vi "VNA Driver Test.vi"() -> ()   [LabVIEW 2011]
uses:
  VNA Command.ctl
  VNA Driver Ref.ctl
panel:
  in  "Tab Control":enum32{"Stimulus", "Measurements"}(tab)=enum."Measurements"
  out "Get Stimulus":T1
  in  "get stimulus":bool
  in  "set stimulus":bool
  in  "Set Stimulus":T1
  in  "mag":bool=TRUE
  out "plot":cluster{dbl, dbl, dbl[][]}(graph)
  in  "S to Meas":enum32{"S11", "S21", "S12", "S22"}[](array[ring])=[enum."S11"]
  in  "measure":bool
  in  "preset":bool
  in  "config":bool
  in  "init":bool
  in  "VNA Drivers":u16(ring) items=["Agilent VNA", "Summitek VNA"]
  in  "load":bool
  in  "stop":bool
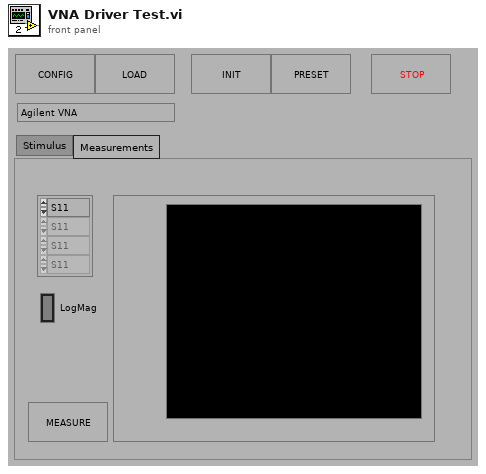
[diagram p1: front panel]
types:
  T1 = cluster{"Use Instrument Settings":bool, "Sweep Type":enum32{"Linear", "Log", "List", "Power", "CW"}, "Sweep":cluster{"Fstart, MHz":dbl, "Fstop, MHz":dbl, "Points":i32}[], "Advanced Settings":bool, "Blank Frequencies":bool, "Power, dBm":dbl, "IFBW, Hz":dbl, "Sweep Time, s":dbl}
  T2 = typedef "VNA Driver Ref.ctl" = refnum<vi>
  T3 = typedef "VNA Command.ctl" = enum16{"LOAD", "INITIALIZE", "PRESET", "GET STIMULUS", "SET STIMULUS", "GET CALIBRATION", "CALIBRATE", "RESTORE", "MEASURE", "RELEASE", "UNLOAD", "CONFIRM", "SORT"}
  T4 = typedef "SP Data.ctl" = cluster{"F0":dbl, "dF":dbl, "Data":cdb[][]}
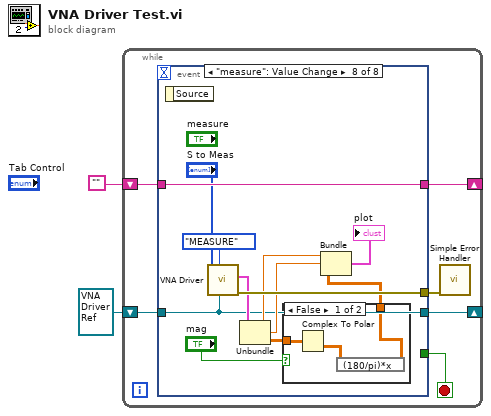
[diagram p0: block diagram]
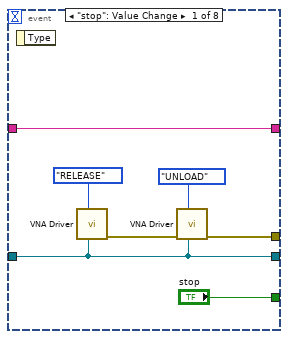
[diagram p2: hidden frame]
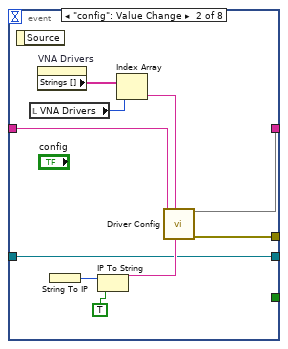
[diagram p3: hidden frame]
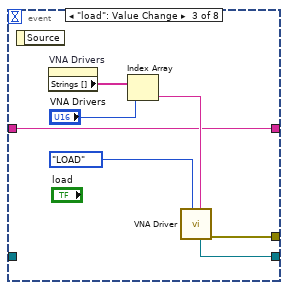
[diagram p4: hidden frame]
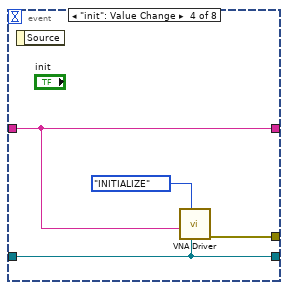
[diagram p5: hidden frame]
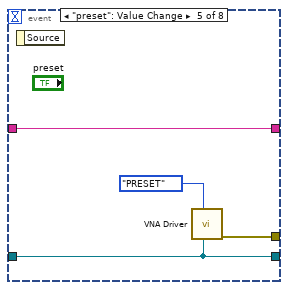
[diagram p6: hidden frame]
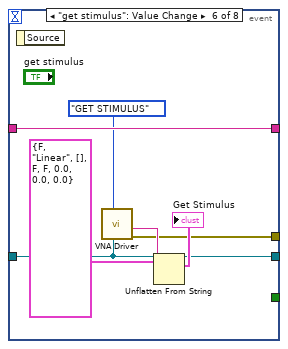
[diagram p7: hidden frame]
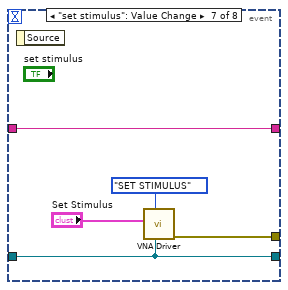
[diagram p8: hidden frame]
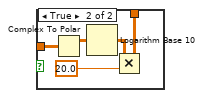
[diagram p9: hidden frame]
diagram:
  n1 = while {
    shift-right: [w6] -> _
    shift-left: "" -> [w5]
    shift-right: [w3] -> _
    shift-left: T2 refnum ("Driver Ref") -> [w4]
    stop <- w8 stop-if-true
    n2 = event shown="[7] \"measure\": Value Change" {
      selector: _ -> [_ _ _ _ _ _ _ _]
      dyn-events: _ -> [_ _ _ _ _ _ _ _]
      timeout: _ -> [_ _ _ _ _ _ _ _]
      tunnel: ["stop" _ _ _ _ _ _ _] -> w8
      tunnel: [w11 w25 w28 w36 w40 w43 w50 w62] -> w7
      tunnel: [w14 w24 w27 w34 w39 w47 w52 w64] -> w6
      tunnel: w5 -> [w14 w23 w27 w34 w39 w47 w52 w64]
      tunnel: w4 -> [w9 w16 _ w33 w37 w41 w48 w53]
      tunnel: [w9 w16 w26 w33 w37 w41 w48 w53] -> w3
      event "stop": Value Change {
        n3 = event-data() -> ()  [unwired: 1 in, 1 out]
        n4 = call "VNA Driver.vi"("Drv Refnum"=w9, "VNA Command"=VNA_Command."RELEASE") -> ("error out"=w12:errorcluster)  [unwired: 5 in, 4 out]
        n5 = call "VNA Driver.vi"("Drv Refnum"=w9, "VNA Command"=VNA_Command."UNLOAD", "error in (no error)"=w12) -> ("error out"=w11:errorcluster)  [unwired: 4 in, 4 out]
      }
      event "config": Value Change {
        n6 = event-data() -> ()  [unwired: 1 in, 1 out]
        n7 = local read "VNA Drivers"() -> (w19:u16)
        n8 = property on="VNA Drivers" class="Ring (strict)"() -> ("Strings []"=w18:string[])  [unwired: 2 in, 2 out]
        n9 = String To IP() -> (0:w22:u32)  [unwired: 1 in]
        n10 = IP To String(1:TRUE, 2:w22) -> (0:w21:string)
        n11 = Index Array(array=w18, index=w19) -> (element=w17:string)
        n12 = call "Driver Config.vi"("CalDue"=w21, "DriverType (\"\")"=w17, "TestStation Client (\"\")"=w23) -> ("error out"=w25:errorcluster, 3:w24)  [unwired: 4 in, 3 out]
      }
      event "load": Value Change {
        n13 = event-data() -> ()  [unwired: 1 in, 1 out]
        n14 = property on="VNA Drivers" class="Ring (strict)"() -> ("Strings []"=w31:string[])  [unwired: 2 in, 2 out]
        n15 = Index Array(array=w31, index="VNA Drivers") -> (element=w29:string)
        n16 = call "VNA Driver.vi"("VNA Driver or\nVNA Configuration (\"\")"=w29, "VNA Command"=VNA_Command."LOAD") -> ("error out"=w28:errorcluster, "dup Drv Refnum"=w26:T2)  [unwired: 5 in, 3 out]
      }
      event "init": Value Change {
        n17 = event-data() -> ()  [unwired: 1 in, 1 out]
        n18 = call "VNA Driver.vi"("Drv Refnum"=w33, "VNA Command"=VNA_Command."INITIALIZE", "Miscellaneous Parameters"=w34) -> ("error out"=w36:errorcluster)  [unwired: 4 in, 4 out]
      }
      event "preset": Value Change {
        n19 = event-data() -> ()  [unwired: 1 in, 1 out]
        n20 = call "VNA Driver.vi"("Drv Refnum"=w37, "VNA Command"=VNA_Command."PRESET") -> ("error out"=w40:errorcluster)  [unwired: 5 in, 4 out]
      }
      event "get stimulus": Value Change {
        n21 = event-data() -> ()  [unwired: 1 in, 1 out]
        n22 = call "VNA Driver.vi"("Drv Refnum"=w41, "VNA Command"=VNA_Command."GET STIMULUS") -> ("error out"=w43:errorcluster, "VNA Flat Output"=w45:string)  [unwired: 5 in, 3 out]
        n23 = Unflatten From String(type=T1 {"Use Instrument Settings"=FALSE, "Sweep Type"=enum."Linear", "Sweep"=[], "Advanced Settings"=FALSE, "Blank Frequencies"=FALSE, "Power, dBm"=0.0, "IFBW, Hz"=0.0, "Sweep Time, s"=0.0} ("Get Stimulus"), binary string=w45) -> (value=→"Get Stimulus":T1)  [unwired: 3 in, 2 out]
      }
      event "set stimulus": Value Change {
        n24 = event-data() -> ()  [unwired: 1 in, 1 out]
        n25 = call "VNA Driver.vi"("Drv Refnum"=w48, "VNA Command"=VNA_Command."SET STIMULUS", "VNA Stimulus"="Set Stimulus") -> ("error out"=w50:errorcluster)  [unwired: 4 in, 4 out]
      }
      event "measure": Value Change {
        n26 = event-data() -> ()  [unwired: 1 in, 1 out]
        n27 = call "VNA Driver.vi"("Drv Refnum"=w53, "VNA Command"=VNA_Command."MEASURE", "Parameters to Measure"="S to Meas") -> ("error out"=w62:errorcluster, "SP Data"=w60:T4)  [unwired: 4 in, 3 out]
        n28 = Unbundle(w60) -> ("F0"=w58:dbl, "dF"=w57:dbl, "Data"=w59:cdb[][])
        n29 = case shown="False" "mag" {
          tunnel: w59 -> [w67 w72]
          tunnel: [w65 w68] -> w56
          frame False {
            n30 = Complex To Polar(r * e^(i*theta)=w67) -> (theta=w66:dbl[][])  [unwired: 1 out]
            n31 = expression code="(180/pi)*x"(w66) -> (w65:dbl[][])
          }
          frame True {
            n32 = Complex To Polar(r * e^(i*theta)=w72) -> (r=w71:dbl[][])  [unwired: 1 out]
            n33 = Logarithm Base 10(1:w71) -> (0:w70:dbl[][])
            n34 = Multiply(x=w70, y=20.0) -> (x*y=w68:dbl[][])
          }
        }
        n35 = Bundle("F0"=w58, "dF"=w57, w56) -> (→"plot":cluster{"F0":dbl, "dF":dbl, dbl[][]})  [unwired: 1 in]
      }
    }
    n36 = call <vilib>:"Simple Error Handler.vi"("error in (no error)"=w7) -> ()  [unwired: 4 in, 5 out]
  }
